vi "Helper SubVI - Compute QRS Duration.vi"(10 "threshold":dbl=-6.8, 11 "valleys":cluster{"locations":dbl[], "amplitudes":dbl[]}) -> (3 "QRS Duration":dbl[](array[numeric]))   [LabVIEW 2023]
doc: "Computes the QRS duration which is the duration between the Q and S waves."
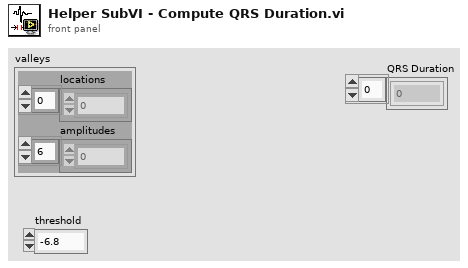
[diagram p1: front panel]
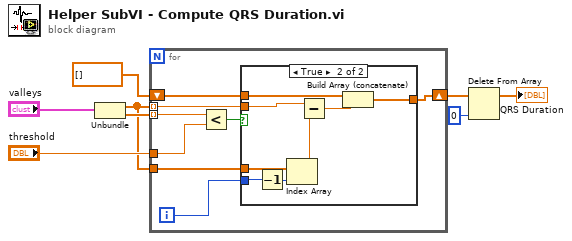
[diagram p0: block diagram]
diagram:
  n1 = Unbundle("valleys") -> ("locations"=w4:dbl[], "amplitudes"=w7:dbl[])
  n2 = for {
    tunnel: w4 -> [w13] mode=indexing
    tunnel: w7 -> [w16] mode=indexing
    tunnel: "threshold" -> [w15]
    shift-right: [w12] -> w3
    shift-left: dbl[] [] -> [w11]
    tunnel: w4 -> [w10]
    i -> [w9]
    n3 = Less?(x=w16, y=w15) -> (x < y?=w14:bool)
    n4 = case shown="True" w14 {
      tunnel: w13 -> [_ w25]
      tunnel: [w17 w24] -> w12
      tunnel: w11 -> [w17 w23]
      tunnel: w10 -> [_ w22]
      tunnel: w9 -> [_ w21]
      frame False {
      }
      frame True {
        n5 = Decrement(x=w21) -> (x-1=w20:i32)
        n6 = Index Array(array=w22, index=w20) -> (element=w18:dbl)
        n7 = Subtract(x=w25, y=w18) -> (x-y=w19:dbl)
        n8 = Build Array (concatenate)(w23, w19) -> (w24:dbl[])
      }
    }
  }
  n9 = Delete From Array(array=w3, index=0) -> (array with subset deleted=→"QRS Duration":dbl[])  [unwired: 1 in, 1 out]
